vi "例4-9.vi"() -> ()   [LabVIEW 2019]
panel:
  out "s":dbl format="%#_4g"
  in  "c":dbl=6.0
  in  "b":dbl=4.0
  in  "a":dbl=3.0
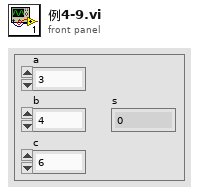
[diagram p1: front panel]
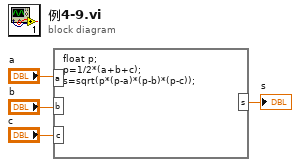
[diagram p0: block diagram]
diagram:
  n1 = formula code="float p;\np=1/2*(a+b+c);\ns=sqrt(p*(p-a)*(p-b)*(p-c));"("a"="a", "b"="b", "c"="c") -> ("s"=→"s":dbl)
